vi "Alm.vi"(8 "error in (no error)":errorcluster caption="错误输入（无错误）", 11 "AllControls Out":T1) -> ()   [LabVIEW 2017]
uses:
  Ctrls/AllControls.ctl
  ComVIS/_OpenG/comparison/comparison.llb/1D Boolean Array Changed__ogtk.vi
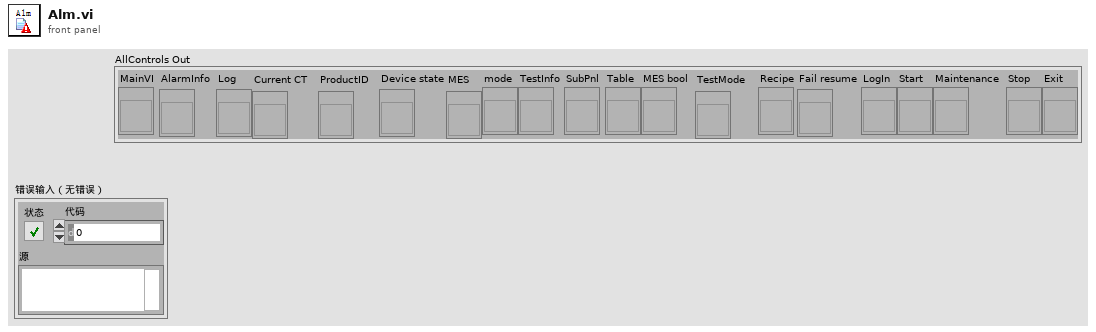
[diagram p1: front panel]
types:
  T1 = typedef "AllControls.ctl" = cluster{"MainVI":refnum<vi>, "AlarmInfo":refnum<vi>, "Log":refnum<vi>, "Current CT":refnum<vi>, "ProductID":refnum<vi>, "Device state":refnum<vi>, "MES":refnum<vi>, "mode":refnum<vi>, "TestInfo":refnum<vi>, "SubPnl":refnum<vi>, "Table":refnum<vi>, "MES bool":refnum<vi>, "TestMode":refnum<vi>, "Recipe":refnum<vi>, "Fail resume":refnum<vi>, "LogIn":refnum<vi>, "Start":refnum<vi>, "Maintenance":refnum<vi>, "Stop":refnum<vi>, "Exit":refnum<vi>}
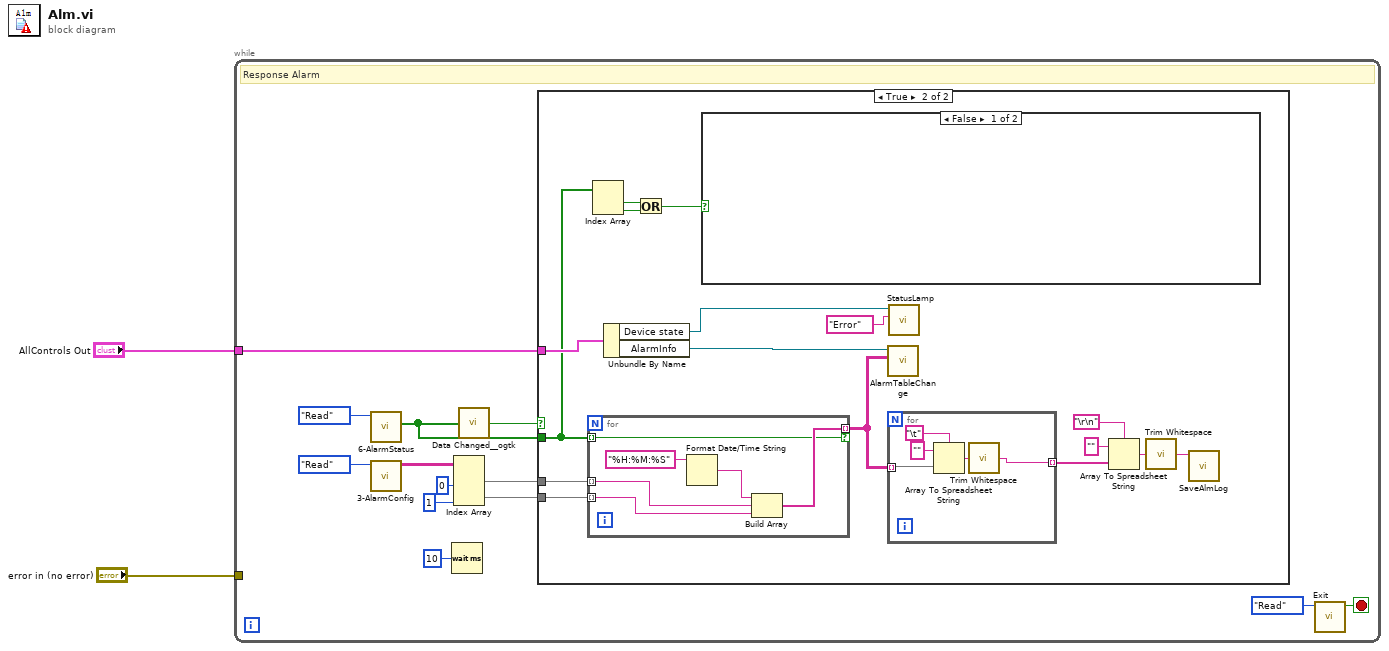
[diagram p0: block diagram]
diagram:
  n1 = while {
    tunnel: "AllControls Out" -> [w12]
    tunnel: "error in (no error)" -> [_]
    stop <- w15 stop-if-true
    # "Response Alarm"
    n2 = call "6-AlarmStatus.vi"("Step"=enum16{"Initial", "Write", "Read"}."Read") -> ("AlarmValue Out"=w4:bool[])  [unwired: 9 in, 1 out]
    n3 = call "3-AlarmConfig.vi"("Step"=enum16{"Initial", "Write", "Read"}."Read") -> ("AlarmConfig Out"=w9:string[][])  [unwired: 9 in, 1 out]
    n4 = Wait (ms)(milliseconds to wait=u32 10 ("等待时间（毫秒）")) -> ()  [unwired: 1 out]
    n5 = Index Array(array=w9, index (col) #1=0 ("禁用的索引 (列)"), index (col) #2=1 ("索引 (列)")) -> (element #1=w6:string[], element #2=w5:string[])  [unwired: 2 in]
    n6 = call-poly "Data Changed__ogtk.vi"("1D Boolean Array"=w4) -> ("Changed"=w3:bool)
    n7 = case shown="True" w3 {
      tunnel: w6 -> [_ w31]
      tunnel: w5 -> [_ w30]
      tunnel: w4 -> [_ w19]
      tunnel: w12 -> [_ w29]
      frame False {
      }
      frame True {
        n8 = for {
          tunnel: w31 -> [w40] mode=indexing
          tunnel: w30 -> [w39] mode=indexing
          tunnel: w19 -> [w37] mode=indexing
          tunnel: [w38] -> w23 mode=indexing if=w37
          n9 = Format Date/Time String(time format string (%c)="%H:%M:%S" ("时间格式字符串(%c)")) -> (date/time string=w41:string)  [unwired: 2 in]
          n10 = Build Array(w41, w40, w39) -> (w38:string[])
        }
        n11 = Index Array(array=w19) -> (element #1=w17:bool, element #2=w18:bool)  [unwired: 2 in]
        n12 = Unbundle By Name(w29) -> ("Device state"=w20:refnum<vi>, "AlarmInfo"=w24:refnum<vi>)
        n13 = Or(x=w17, y=w18) -> (x .or. y?=w16:bool)
        n14 = case shown="False" w16 {
          frame False {
          }
          frame True {
          }
        }
        n15 = call "AlarmTableChange.vi"("AlarmData"=w23, "AlarmInfo"=w24) -> ()  [unwired: 9 in, 1 out]
        n16 = for {
          tunnel: w23 -> [w36] mode=indexing
          tunnel: [w32] -> w26 mode=indexing
          n17 = Array To Spreadsheet String(delimiter (Tab)="\t", array=w36, 3:"" ("format string")) -> (spreadsheet string=w33:string)
          n18 = call <vilib>:"Trim Whitespace.vi"("string"=w33) -> ("trimmed string"=w32:string)  [unwired: 1 in]
        }
        n19 = call "StatusLamp.vi"("State"="Error", "Boolean输入"=w20) -> ()  [unwired: 9 in, 1 out]
        n20 = Array To Spreadsheet String(delimiter (Tab)="\r\n", array=w26, 3:"" ("format string")) -> (spreadsheet string=w25:string)
        n21 = call <vilib>:"Trim Whitespace.vi"("string"=w25) -> ("trimmed string"=w22:string)  [unwired: 1 in]
        n22 = call "SaveAlmLog.vi"("AlmLog"=w22) -> ()  [unwired: 10 in, 1 out]
      }
    }
    n23 = call "Exit.vi"("Step"=enum16{"Initial", "Write", "Read"}."Read" ("step")) -> ("Exit Out"=w15:bool)  [unwired: 9 in, 1 out]
  }
